vi "Destroy event.vi"(8 "error in (no error)":errorcluster, 11 "Measurement gg in":refnum<class "Measurement gg.lvclass">) -> (0 "error out":errorcluster, 3 "Measurement gg out":refnum<class "Measurement gg.lvclass">)   [LabVIEW 2020, in "Measurement gg.lvlib" / "Measurement gg.lvclass"]
uses:
  Measurement gg.lvclass
  Measurement gg.lvclass/Measurement gg.ctl
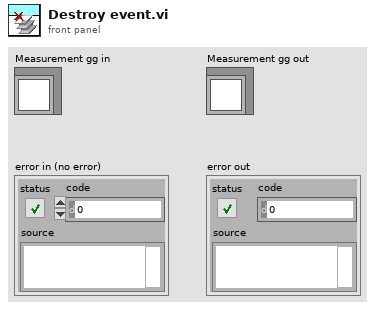
[diagram p1: front panel]
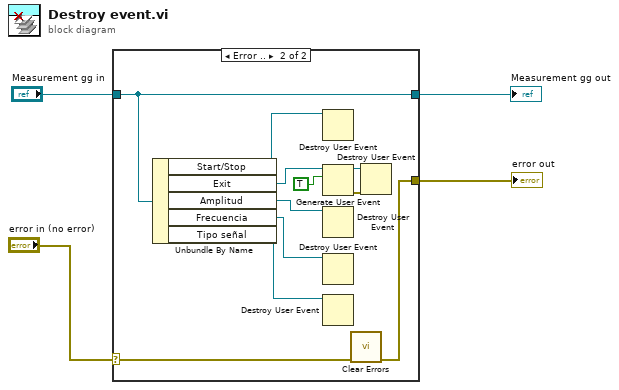
[diagram p0: block diagram]
diagram:
  n1 = case shown="Error .." "error in (no error)" {
    selector: "error in (no error)" -> [w6 w16]
    tunnel: [w6 w15] -> w2
    tunnel: [w5 w17] -> w3
    tunnel: "Measurement gg in" -> [w5 w17]
    frame No Error {
    }
    frame Error {
      n2 = Unbundle By Name(w17) -> ("Start/Stop"=w14:refnum<user-event>, "Exit"=w13:refnum<user-event>, "Amplitud"=w10:refnum<user-event>, "Frecuencia"=w9:refnum<user-event>, "Tipo señal"=w8:refnum<user-event>)
      n3 = Destroy User Event(user event=w14) -> ()  [unwired: 1 in, 1 out]
      n4 = Generate User Event(user event=w13, event data cluster=TRUE ("event data")) -> (user event out=w12:refnum<user-event>, error out=w11:errorcluster)  [unwired: 2 in]
      n5 = Destroy User Event(user event=w10) -> ()  [unwired: 1 in, 1 out]
      n6 = Destroy User Event(user event=w9) -> ()  [unwired: 1 in, 1 out]
      n7 = Destroy User Event(user event=w8) -> ()  [unwired: 1 in, 1 out]
      n8 = call <vilib>:"Clear Errors.vi"("error in (no error)"=w16) -> ("error out"=w15:errorcluster)  [unwired: 5 in, 1 out]
      n9 = Destroy User Event(user event=w12, error in=w11) -> ()  [unwired: 1 out]
    }
  }
  "Measurement gg out" <- w3
  "error out" <- w2
